vi "DSF.Engine.Transfer Group.Initialize.vi"(8 "error in (no error)":errorcluster, 9 "Transfers":refnum<class "DSF.Engine.Transfer.lvclass">[](array[class]), 10 "Configuration":refnum<class "DSF.Shared.Configuration.Transfer Group.lvclass">, 11 "Transfer Group type":refnum<class "DSF.Engine.Transfer Group.lvclass">) -> (0 "error out":errorcluster, 3 "Transfer Group out":refnum<class "DSF.Engine.Transfer Group.lvclass">)   [LabVIEW 2016, in "DSF.Engine.lvlib" / "DSF.Engine.Transfer Group.lvclass"]
uses:
  DSF.Engine.Transfer Group.lvclass
  Shared/Classes/Transfer Group/DSF.Shared.Configuration.Transfer Group.lvclass
  DSF.Engine.Transfer.lvclass
  Shared/Classes/Transfer Group/DSF.Shared.Configuration.Transfer Group.lvclass/DSF.Shared.Configuration.Transfer Group.ctl
  DSF.Engine.Transfer Group.lvclass/DSF.Engine.Transfer Group.ctl
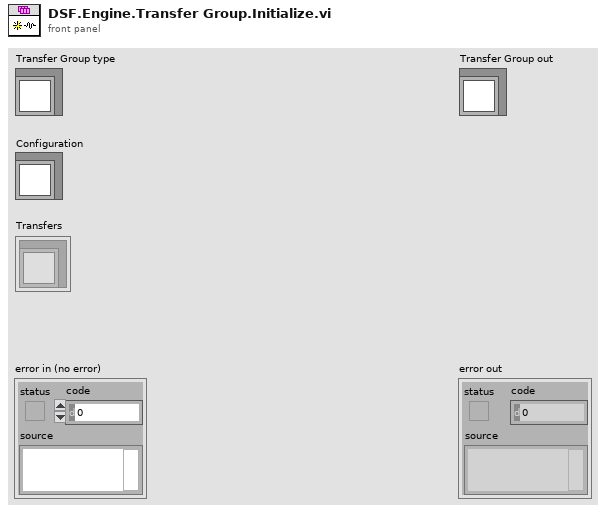
[diagram p1: front panel]
types:
  T1 = typedef "DSF.Shared.lvlib/DSF.Shared.Typedefs.Direction.ctl" = enum16{"Tx", "Rx"}
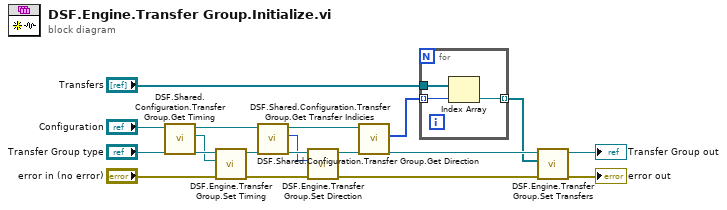
[diagram p0: block diagram]
diagram:
  n1 = call "DSF.Shared.Configuration.Transfer Group.Get Timing.vi"("Transfer Group Configuration in"="Configuration") -> ("Timing"=w11:refnum<class "DSF.Engine.Timing.lvclass">, "Transfer Group Configuration out"=w10:refnum<class "DSF.Shared.Configuration.Transfer Group.lvclass">)  [unwired: 9 in]
  n2 = call "DSF.Engine.Transfer Group.Set Timing.vi"("Timing"=w11, "Transfer Group in"="Transfer Group type") -> ("Transfer Group out"=w9:refnum<class "DSF.Engine.Transfer Group.lvclass">)  [unwired: 9 in]
  n3 = call "DSF.Shared.Configuration.Transfer Group.Get Direction.vi"("Transfer Group Configuration in"=w10) -> ("Direction"=w8:T1, "Transfer Group Configuration out"=w7:refnum<class "DSF.Shared.Configuration.Transfer Group.lvclass">)  [unwired: 9 in]
  n4 = call "DSF.Engine.Transfer Group.Set Direction.vi"("Direction"=w8, "Transfer Group in"=w9) -> ("Transfer Group out"=w4:refnum<class "DSF.Engine.Transfer Group.lvclass">)  [unwired: 9 in]
  n5 = call "DSF.Shared.Configuration.Transfer Group.Get Transfer Indicies.vi"("Transfer Group Configuration in"=w7) -> ("Transfer indices"=w6:i32[])  [unwired: 9 in, 1 out]
  n6 = for {
    tunnel: w6 -> [w15] mode=indexing
    tunnel: "Transfers" -> [w16]
    tunnel: [w14] -> w3 mode=indexing
    n7 = Index Array(array=w16, index=w15) -> (element=w14:refnum<class "DSF.Engine.Transfer.lvclass">)
  }
  n8 = call "DSF.Engine.Transfer Group.Set Transfers.vi"("Transfers"=w3, "Transfer Group in"=w4) -> ("Transfer Group out"=→"Transfer Group out":refnum<class "DSF.Engine.Transfer Group.lvclass">)  [unwired: 9 in]
  "error out" <- "error in (no error)"
